vi "CD Read Engine.vi"(7 "Error (in)":errorcluster, 8 "Output Channel Data []":T1[](array[typedef]) {"Labels Settings"."Label" format="%.0o"}, 9 "Card Parameters (in)":T16, 10 "Data (in)":dbl[](array[numeric])) -> (0 "Error (out)":errorcluster, 3 "Data (out)":dbl[](array[numeric]))   [LabVIEW 2017, in "Ballard Arinc-429 Engine.lvlib"]
uses:
  Ballard Arinc-429 Engine.lvlib
  <instrlib>/BTICardLib/Public/Controls/429 Record.ctl
  <instrlib>/BTICardLib/Public/Controls/Seq Run Status.ctl
  <instrlib>/BTICardLib/Public/Controls/Seq Fill Status.ctl
  RT Controls/RT HW Channel.ctl
  RT Controls/RT Label Settings.ctl
  Shared/Controls and Global/Label.ctl
  Shared/Controls and Global/transferPeriod.ctl
  RT Controls/Driver Data.ctl
  RT Controls/RT Word Settings.ctl
  <vilib>/NI Veristand/Custom Device API/Block Data Reference.ctl
  <vilib>/NI Veristand/Custom Device API/Data Reference.ctl
  RT Controls/RT Param Setting.ctl
  Shared/Controls and Global/Start Bit.ctl
  Shared/Controls and Global/Number of Bits.ctl
  Shared/Controls and Global/TransferType.ctl
  RT Controls/Card Parameters.ctl
  <instrlib>/BTICardLib/BTICardLV.lvlib
  Shared/Ballard Arinc-429 Shared.lvlib
  <vilib>/NI Veristand/Custom Device API/Custom Device API.lvlib
panel:
  in  "Tab Control":enum32{"Controls & Indicators", "Misc"}(tab)
  out "# of records read":i32
  out "Record []":T13[](array[typedef]) {"type" format="%04x"; "timestamp" format="%08x"; "msgact" format="%04x"; "data" format="%08x"; "timestamph" format="%08x"}
  out "run status":T14 items=["SEQ_STARTED", "SEQ_STOPPED", "SEQ_ERROR"]
  out "fill status":T15 items=["SEQ_EMPTY", "SEQ_PARTIAL", "SEQ_FULL"]
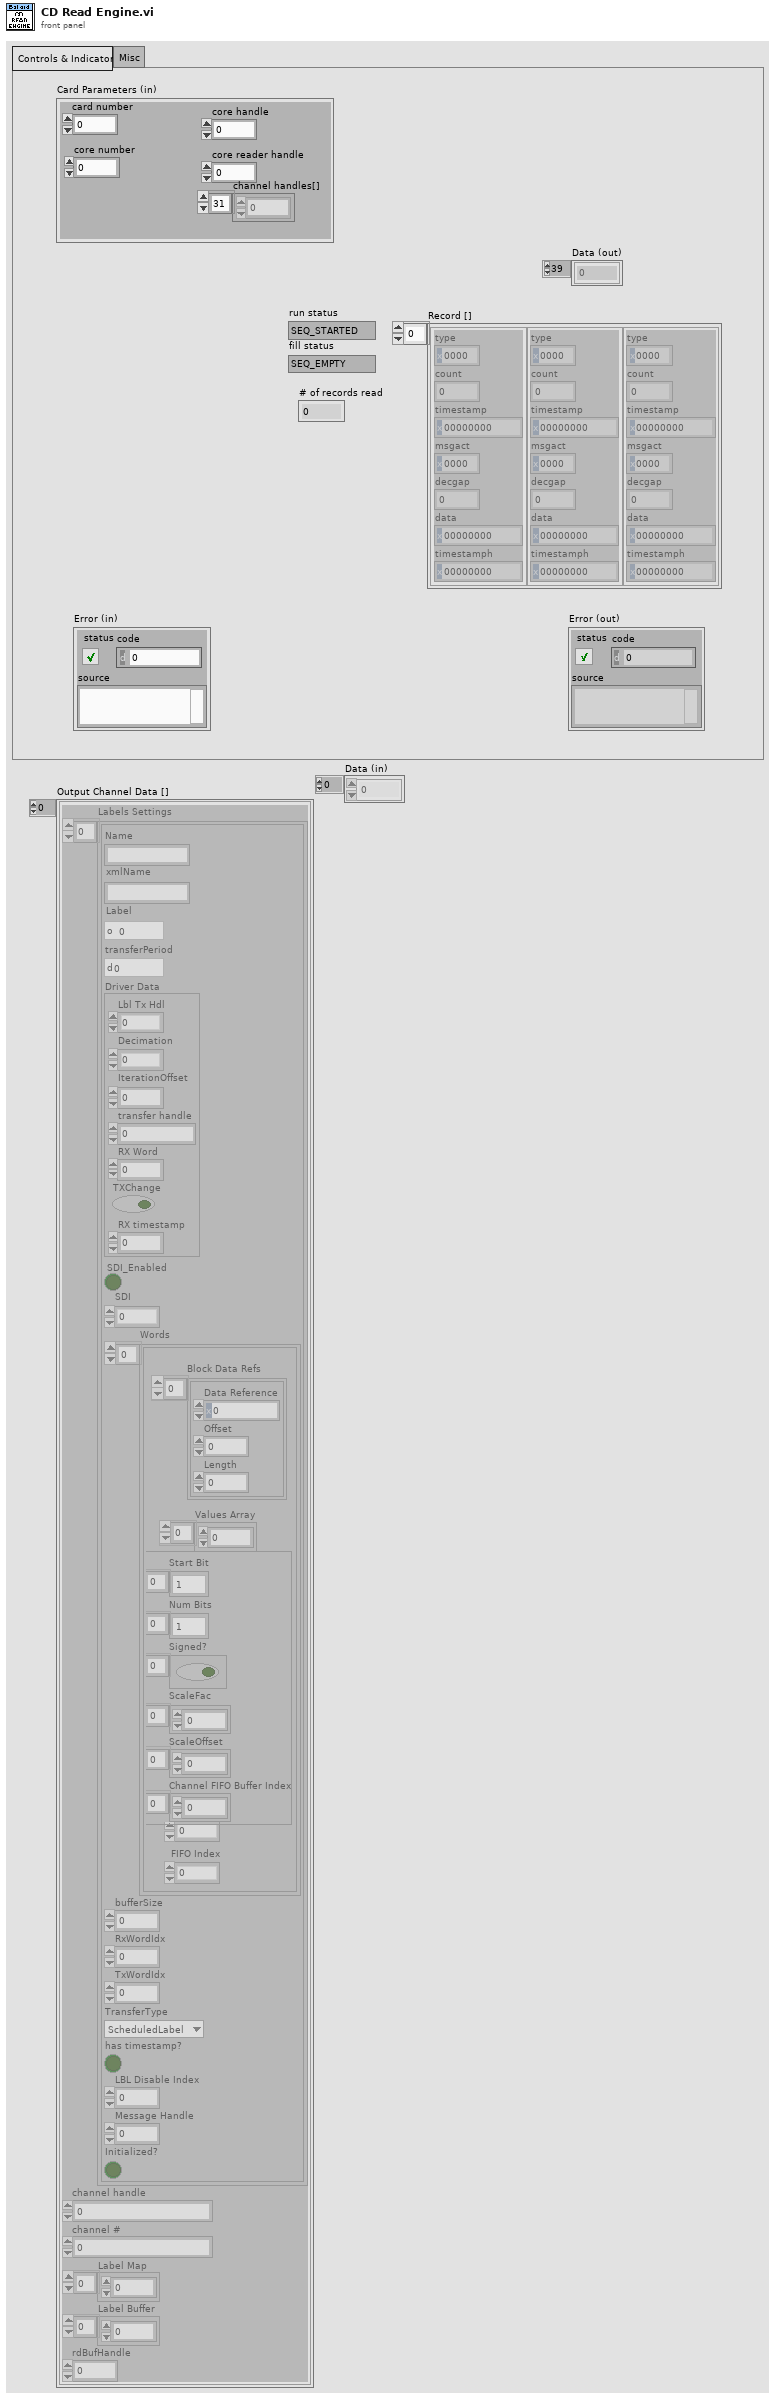
[diagram p1: front panel]
types:
  T1 = typedef "Ballard Arinc-429 Engine.lvlib/RT HW Channel.ctl" = cluster{"Labels Settings":T2[], "channel handle":u32, "channel #":u16, "Label Map":i32[], "Label Buffer":u32[], "rdBufHandle":u32}
  T2 = typedef "Ballard Arinc-429 Engine.lvlib/RT Label Settings.ctl" = cluster{"Name":string, "xmlName":string, "Label":T3, "transferPeriod":T4, "Driver Data":T5, "SDI_Enabled":bool, "SDI":u8, "Words":T6[], "bufferSize":u32, "RxWordIdx":i32, "TxWordIdx":i32, "TransferType":T12, "has timestamp?":bool, "LBL Disable Index":i32, "Message Handle":u64, "Initialized?":bool}
  T3 = typedef "Ballard Arinc-429 Shared.lvlib/Label.ctl" = u8
  T4 = typedef "Ballard Arinc-429 Shared.lvlib/transferPeriod.ctl" = u32
  T5 = typedef "Ballard Arinc-429 Engine.lvlib/Driver Data.ctl" = cluster{"Lbl Tx Hdl":u32, "Decimation":i32, "IterationOffset":i32, "transfer handle":u32, "RX Word":u32, "TXChange":bool, "RX timestamp":dbl}
  T6 = typedef "Ballard Arinc-429 Engine.lvlib/RT Word Settings.ctl" = cluster{"Block Data Refs":T7[], "Values Array":dbl[], "Length":i32, "FIFO Index":i32, "Param Setting":T9}
  T7 = typedef "Custom Device API.lvlib/Block Data Reference.ctl" = cluster{"Data Reference":T8, "Offset":u64, "Length":u64}
  T8 = typedef "Custom Device API.lvlib/Data Reference.ctl" = i32
  T9 = typedef "Ballard Arinc-429 Engine.lvlib/RT Param Setting.ctl" = cluster{"Start Bit":T10[], "Num Bits":T11[], "Signed?":bool[], "ScaleFac":dbl[], "ScaleOffset":dbl[], "Channel FIFO Buffer Index":i32[]}
  T10 = typedef "Ballard Arinc-429 Shared.lvlib/Start Bit.ctl" = i32
  T11 = typedef "Ballard Arinc-429 Shared.lvlib/Number of Bits.ctl" = i32
  T12 = typedef "Ballard Arinc-429 Shared.lvlib/TransferType.ctl" = enum16{"ScheduledLabel", "Acyclic", "Block", "Strobe"}
  T13 = typedef "BTICardLV.lvlib/429 Record.ctl" = cluster{"type":u16, "count":u16, "timestamp":u32, "msgact":u16, "decgap":u16, "data":u32, "timestamph":u32}
  T14 = typedef "BTICardLV.lvlib/Seq Run Status.ctl" = u32
  T15 = typedef "BTICardLV.lvlib/Seq Fill Status.ctl" = u32
  T16 = typedef "Ballard Arinc-429 Engine.lvlib/Card Parameters.ctl" = cluster{"card number":i32, "core number":i32, "core handle":u64, "core reader handle":u64, "channel handles[]":u64[]}
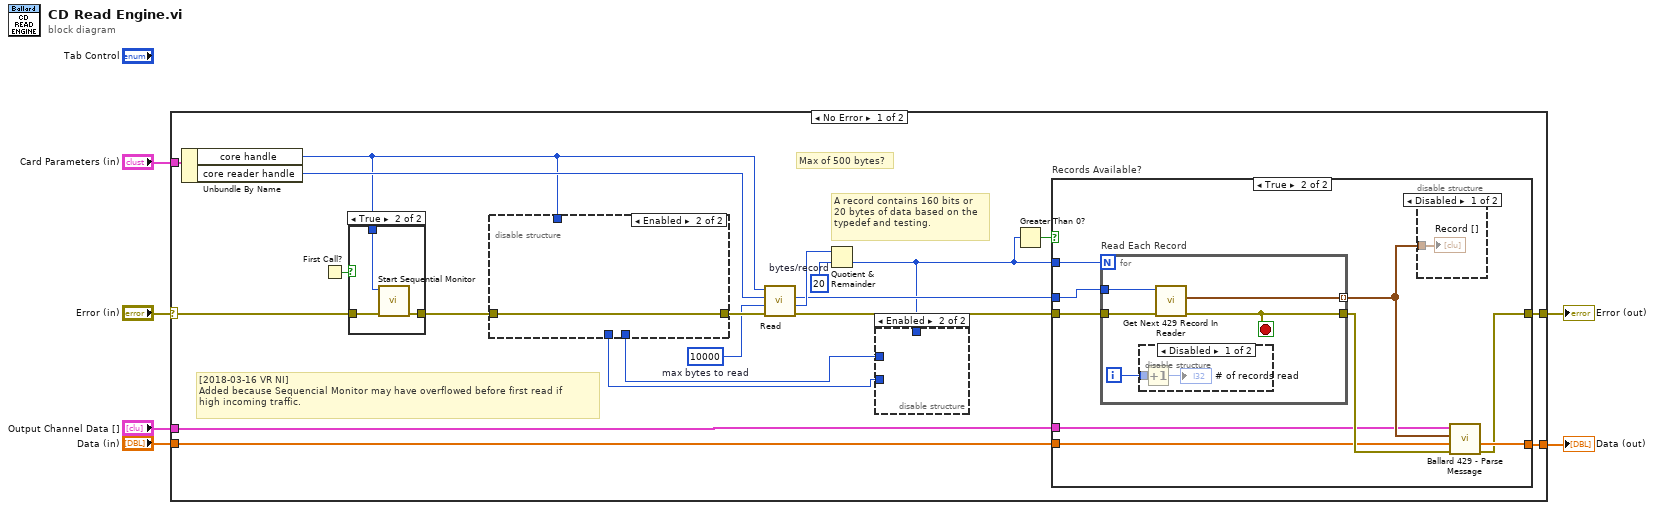
[diagram p0: block diagram]
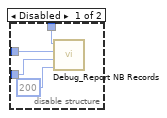
[diagram p3: hidden frame]
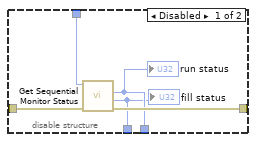
[diagram p4: hidden frame]
diagram:
  n1 = case shown="No Error" "Error (in)" {
    selector: "Error (in)" -> [w9 w61]
    tunnel: "Card Parameters (in)" -> [w18 _]
    tunnel: "Output Channel Data []" -> [w17 _]
    tunnel: [w16 w60] -> w4
    tunnel: [w15 w61] -> w3
    tunnel: "Data (in)" -> [w14 w60]
    frame No Error {
      w22 = 20  # bytes/record
      w24 = 10000  # max bytes to read
      # "[2018-03-16 VR NI]\nAdded because Sequencial Monitor may have overflowed before first read if\nhigh incoming traffic."
      # "A record contains 160 bits or 20 bytes of data based on the typedef and testing."
      # "Max of 500 bytes?"
      n2 = Unbundle By Name(w18) -> ("core handle"=w10:u64, "core reader handle"=w26:u64)
      n3 = First Call?() -> (First Call?: T/F=w7:bool)
      n4 = case shown="True" w7 {
        tunnel: w10 -> [_ w30]
        tunnel: w9 -> [w27 w29]
        tunnel: [w27 w28] -> w8
        frame False {
        }
        frame True {
          n5 = call <instrlib>:"Start Sequential Monitor.vi"("error in (no error)"=w29, "core handle in"=w30) -> ("error out"=w28:errorcluster)  [unwired: 8 in, 1 out]
        }
      }
      n6 = disable-structure shown="Enabled" {
        disable-tunnel: w10 -> [w39 _]
        disable-tunnel: w8 -> [w38 w40]
        disable-tunnel: [w37 w40] -> w25
        disable-tunnel: [w36 _] -> w12
        disable-tunnel: [w35 _] -> w11
        frame Disabled {
          n7 = call <instrlib>:"Get Sequential Monitor Status.vi"("error in (no error)"=w38, "core handle in"=w39) -> ("error out"=w37:errorcluster, "fill status"=w35:T15, "run status"=w36:T14)  [unwired: 6 in, 1 out]
          "run status" <- w36
          "fill status" <- w35
        }
        frame Enabled {
        }
      }
      n8 = call <instrlib>:"Read.vi"("error in (no error)"=w25, "max bytes to read"=w24, "core reader handle in"=w26, "core handle in"=w10) -> ("error out"=w19:errorcluster, "bytes read"=w23:i32, "core reader handle out"=w20:u64)  [unwired: 4 in, 1 out]
      n9 = Quotient & Remainder(x=w23, y=w22) -> (floor(x/y)=w13:i32)  [unwired: 1 out]
      n10 = disable-structure shown="Enabled" {
        disable-tunnel: w13 -> [w34 _]
        disable-tunnel: w12 -> [w32 _]
        disable-tunnel: w11 -> [w31 _]
        frame Disabled {
          n11 = call "Debug_Report NB Records.vi"("Decimation"=200, "fill status"=w31, "run status"=w32, "NB of Records Available"=w34) -> ()  [unwired: 8 in]
        }
        frame Enabled {
        }
      }
      n12 = Greater Than 0?(x=w13) -> (x > 0?=w21:bool)
      n13 = case "Records Available?" shown="True" w21 {
        tunnel: w19 -> [w42 w51]
        tunnel: [w42 w44] -> w15
        tunnel: w20 -> [_ w50]
        tunnel: w13 -> [_ w49]
        tunnel: w17 -> [_ w46]
        tunnel: [w41 w45] -> w16
        tunnel: w14 -> [w41 w43]
        frame False {
        }
        frame True {
          n14 = for "Read Each Record" {
            N: w49 -> [_]
            tunnel: w50 -> [w56]
            tunnel: w51 -> [w57]
            tunnel: [w54] -> w47 mode=indexing
            tunnel: [w53] -> w48
            i -> [w55]
            stop <- w53 stop-if-true
            n15 = disable-structure shown="Disabled" {
              disable-tunnel: w55 -> [w59 _]
              frame Disabled {
                n16 = Increment(x=w59) -> (x+1=→"# of records read":i32)
              }
              frame Enabled {
              }
            }
            n17 = call <instrlib>:"Get Next 429 Record In Reader.vi"("error in (no error)"=w57, "core reader handle in"=w56) -> ("error out"=w53:errorcluster, "record out"=w54:T13)  [unwired: 7 in, 1 out]
          }
          n18 = disable-structure shown="Disabled" {
            disable-tunnel: w47 -> [w52 _]
            frame Disabled {
              "Record []" <- w52
            }
            frame Enabled {
            }
          }
          n19 = call "Ballard 429 - Parse Message.vi"("Error (in)"=w48, "Data (in)"=w43, "Record []"=w47, "Channel Data []"=w46) -> ("Error (out)"=w44:errorcluster, "Doubles []"=w45:dbl[])  [unwired: 6 in]
        }
      }
    }
    frame Error {
    }
  }
  "Error (out)" <- w3
  "Data (out)" <- w4
